vi "find_rects.vi"(5 "shrinkFactor":i32=1, 6 "Field of View":cluster{"fieldOfViewX":sgl, "fieldOfViewY":sgl}, 7 "logFileDir":string, 8 "error in":errorcluster, 9 "debug":bool, 10 "find_patches parameters":T2, 11 "Image":T3) -> (0 "error out":errorcluster, 2 "rects":T1(array[cluster]))   [LabVIEW 2017, in "Vision.lvlib"]
uses:
  Vision.lvlib
  <vilib>/vision/Image Controls.llb/IMAQ Image.ctl
  find_rects_parameters.ctl
  bin/Vision.dll
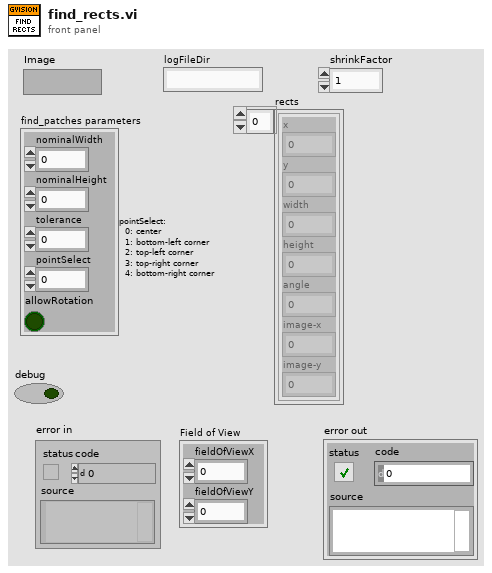
[diagram p1: front panel]
types:
  T1 = cluster{"x":dbl, "y":dbl, "width":dbl, "height":dbl, "angle":dbl, "image-x":dbl, "image-y":dbl}[]
  T2 = typedef "Vision.lvlib/find_rects_parameters.ctl" = cluster{"nominalWidth":sgl, "nominalHeight":sgl, "tolerance":sgl, "pointSelect":sgl, "allowRotation":bool}
  T3 = typedef "IMAQ Image.ctl" = refnum<image>
  T4 = enum32{"Map Pixel Pointer", "Unmap Pixel Pointer", "Get Pixels Infos"}
  T5 = cluster{"x":dbl, "y":dbl, "width":dbl, "height":dbl, "angle":dbl, "image-x":dbl, "image-y":dbl}
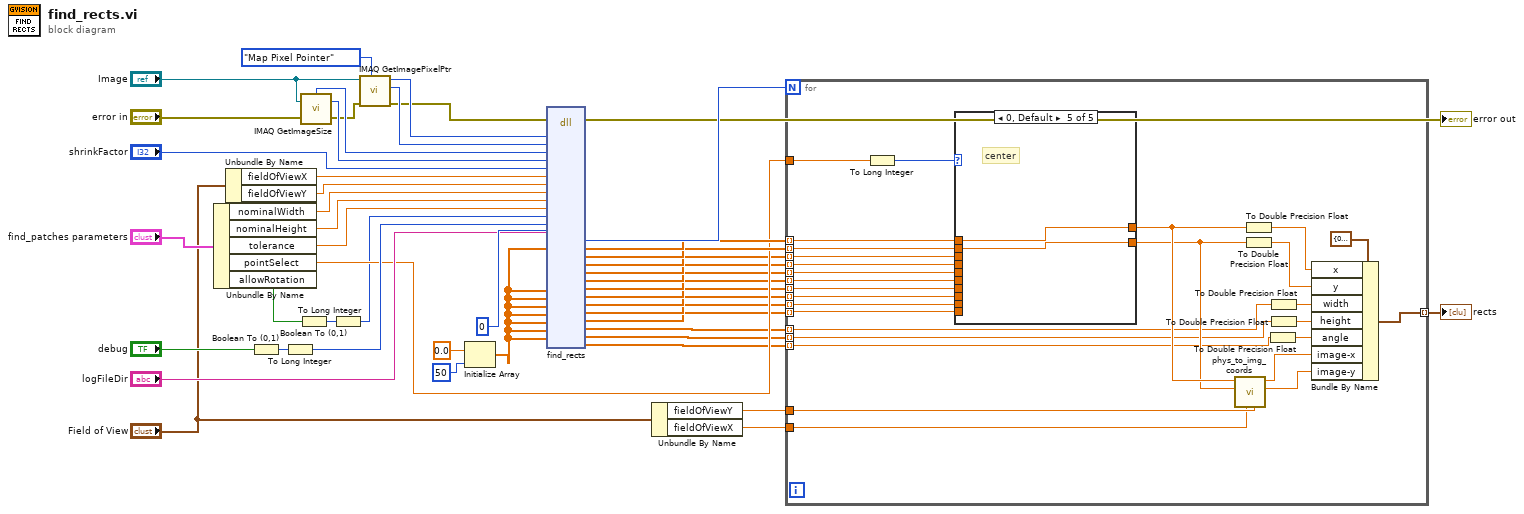
[diagram p0: block diagram]
diagram:
  n1 = Unbundle By Name("find_patches parameters") -> ("nominalWidth"=w31:sgl, "nominalHeight"=w30:sgl, "tolerance"=w29:sgl, "pointSelect"=w16:sgl, "allowRotation"=w1:bool)
  n2 = Unbundle By Name("Field of View") -> ("fieldOfViewX"=w34:sgl, "fieldOfViewY"=w33:sgl)
  n3 = Boolean To (0,1)(Boolean="debug") -> (0, 1=w27:i16)
  n4 = To Long Integer(number=w27) -> (32bit integer=w26:i32)
  n5 = Boolean To (0,1)(Boolean=w1) -> (0, 1=w3:i16)
  n6 = call "IMAQ GetImageSize"("Image"="Image", "error in (no error)"="error in") -> ("Y Resolution"=w43:i32, "X Resolution"=w44:i32, "error out"=w37:errorcluster)  [unwired: 2 in]
  n7 = To Long Integer(number=w3) -> (32bit integer=w2:i32)
  n8 = call "IMAQ GetImagePixelPtr"("Function"=T4."Map Pixel Pointer", "error in (no error)"=w37, "Image"="Image") -> ("error out"=w36:errorcluster, "LineWidth(Pixels)"=w45:i32, "Pixel Pointer out"=w46:u64)  [unwired: 3 in, 3 out]
  n9 = Initialize Array(sgl 0.0 ("element"), 50 ("dimension size")) -> (w15:sgl[])
  n10 = dll-call lib="C:/Users/Caleb/Desktop/nebraska-silicon-lab/pixel-gantry-extra/LV/bin/Vision.dll" fn="find_rects"(error in=w36, "imgPtr"=w46, "imgLineWidth"=w45, "imgWidth"=w44, "imgHeight"=w43, "shrinkFactor"="shrinkFactor", "fieldOfViewX"=w34, "fieldOfViewY"=w33, "nominalWidth"=w31, "nominalHeight"=w30, "tolerance"=w29, "allowRotation"=w2, "debug"=w26, "logFileDir"="logFileDir", "Nrects"=0, "rectXCenters"=w15, "rectYCenters"=w15, "rectXBLCorners"=w15, "rectYBLCorners"=w15, "rectXTLCorners"=w15, "rectYTLCorners"=w15, "rectXTRCorners"=w15, "rectYTRCorners"=w15, "rectXBRCorners"=w15, "rectYBRCorners"=w15, "rectWidths"=w15, "rectHeights"=w15, "rectAngles"=w15) -> (error out=→"error out":errorcluster, "Nrects"=w21:i32, "rectXCenters"=w20:sgl[], "rectYCenters"=w19:sgl[], "rectXBLCorners"=w11:sgl[], "rectYBLCorners"=w10:sgl[], "rectXTLCorners"=w9:sgl[], "rectYTLCorners"=w8:sgl[], "rectXTRCorners"=w7:sgl[], "rectYTRCorners"=w6:sgl[], "rectXBRCorners"=w5:sgl[], "rectYBRCorners"=w4:sgl[], "rectWidths"=w12:sgl[], "rectHeights"=w13:sgl[], "rectAngles"=w14:sgl[])  [unwired: 16 in, 1 out]
  n11 = Unbundle By Name("Field of View") -> ("fieldOfViewY"=w24:sgl, "fieldOfViewX"=w23:sgl)
  n12 = for {
    N: w21 -> [_]
    tunnel: w20 -> [w66] mode=indexing
    tunnel: w19 -> [w65] mode=indexing
    tunnel: [w75] -> w17 mode=indexing
    tunnel: w24 -> [w62]
    tunnel: w23 -> [w61]
    tunnel: w13 -> [w58] mode=indexing
    tunnel: w16 -> [w59]
    tunnel: w14 -> [w57] mode=indexing
    tunnel: w12 -> [w56] mode=indexing
    tunnel: w11 -> [w55] mode=indexing
    tunnel: w10 -> [w54] mode=indexing
    tunnel: w9 -> [w53] mode=indexing
    tunnel: w8 -> [w52] mode=indexing
    tunnel: w7 -> [w51] mode=indexing
    tunnel: w6 -> [w50] mode=indexing
    tunnel: w5 -> [w49] mode=indexing
    tunnel: w4 -> [w48] mode=indexing
    n13 = To Long Integer(number=w59) -> (32bit integer=w60:i32)
    n14 = case shown="0, Default" w60 {
      tunnel: w66 -> [_ _ _ _ w85]
      tunnel: w65 -> [_ _ _ _ w84]
      tunnel: [w77 w79 w81 w83 w85] -> w64
      tunnel: [w76 w78 w80 w82 w84] -> w63
      tunnel: w55 -> [w77 _ _ _ _]
      tunnel: w54 -> [w76 _ _ _ _]
      tunnel: w53 -> [_ w79 _ _ _]
      tunnel: w52 -> [_ w78 _ _ _]
      tunnel: w51 -> [_ _ w81 _ _]
      tunnel: w50 -> [_ _ w80 _ _]
      tunnel: w49 -> [_ _ _ w83 _]
      tunnel: w48 -> [_ _ _ w82 _]
      frame 1 {
        # "bottom-left"
      }
      frame 2 {
        # "top-left"
      }
      frame 3 {
        # "top-right"
      }
      frame 4 {
        # "bottom-right"
      }
      frame 0, Default {
        # "center"
      }
    }
    n15 = call "phys_to_img_coords.vi"("fov_y"=w62, "fov_x"=w61, "y"=w63, "x"=w64) -> ("image_y"=w70:dbl, "image_x"=w71:dbl)  [unwired: 6 in]
    n16 = To Double Precision Float(number=w64) -> (double precision float=w74:dbl)
    n17 = To Double Precision Float(number=w63) -> (double precision float=w73:dbl)
    n18 = To Double Precision Float(number=w57) -> (double precision float=w67:dbl)
    n19 = To Double Precision Float(number=w56) -> (double precision float=w72:dbl)
    n20 = To Double Precision Float(number=w58) -> (double precision float=w69:dbl)
    n21 = Bundle By Name(cluster=T5 {"x"=0.0, "y"=0.0, "width"=0.0, "height"=0.0, "angle"=0.0, "image-x"=0.0, "image-y"=0.0}, "x"=w74, "y"=w73, "width"=w72, "height"=w69, "angle"=w67, "image-x"=w71, "image-y"=w70) -> (w75:T5)
  }
  "rects" <- w17
